vi "CONSTANT - VIP API Version.vi"() -> (2 "Version":string="1.0.0.0")   [LabVIEW 2011, in "G CLI VIP.lvlib"]
uses:
  G CLI VIP.lvlib
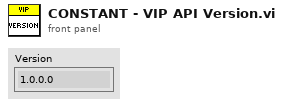
[diagram p1: front panel]
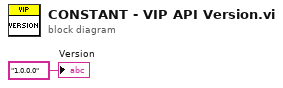
[diagram p0: block diagram]
diagram:
  "Version" <- "1.0.0.0"
